vi "Main.vi"(8 "error in":errorcluster, 11 "Controller in":refnum<class "Controller.lvclass">) -> (0 "error out":errorcluster, 3 "Controller out":refnum<class "Controller.lvclass">)   [LabVIEW 2024, in "Controller.lvclass"]
doc: "The <b>Queued Message Handler</b> of the Worker that owns this VI."
uses:
  Controller.lvclass
  Controller.lvclass/Controller.ctl
  Initialization Data.ctl
  Response Cases.ctl
  <vilib>/addons/_Workers/Library/Case Label.ctl
  <vilib>/addons/_Workers/Library/Workers.lvlib
  rqp_Receive CPU Precent.ctl
  CPU Percent/CPU Percent.lvclass
  Place Temperature/Place Temperature.lvclass
  Place Temperature/rqp_Set Place.ctl
  rqp_Receive Temperature.ctl
  Report/Report.lvclass
  Report/rqp_Receive Log Interval.ctl
  rwr_Get Actual Data Reply.ctl
  C:/Program Files (x86)/National Instruments/LabVIEW 2024/vi.lib/addons/_Workers/Library/Classes/Worker/Worker.lvclass
  BEEP/BEEP.lvclass
panel:
  in  "Log Interval [ms]":i32=2000
  in  "bShowCSV":bool
  in  "Places":string(combo)="Baden, CH"
  out "Temperature":dbl(graph)
  out "Percentage":dbl(graph)
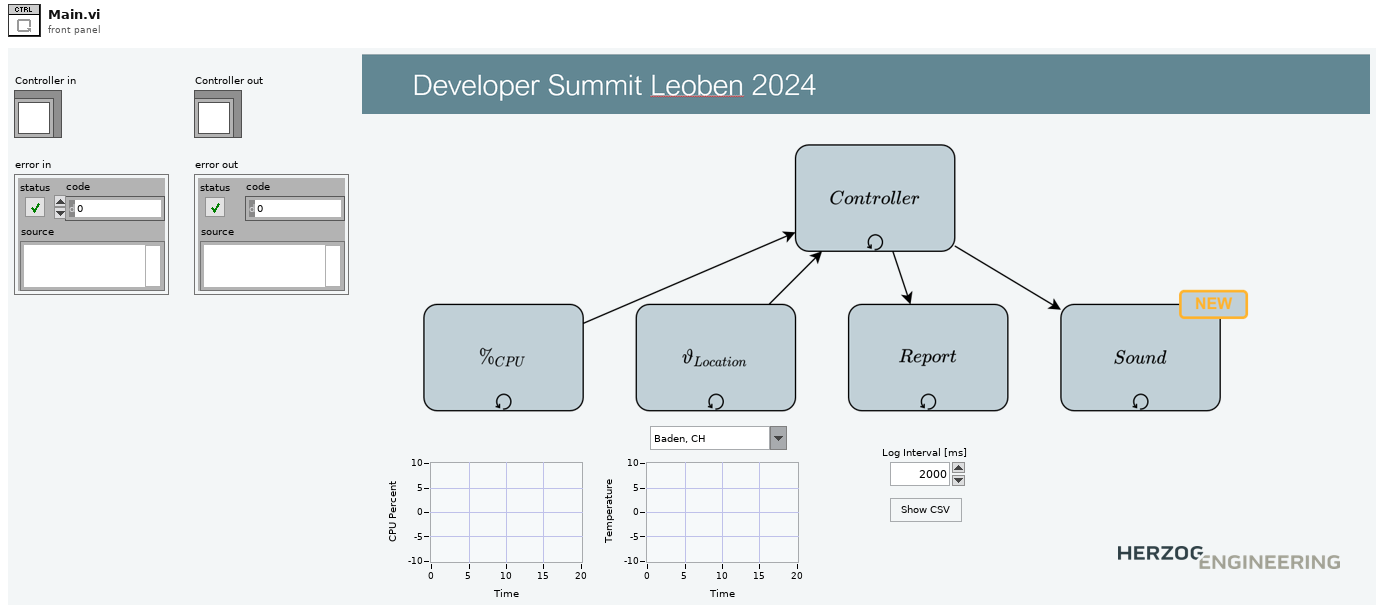
[diagram p1: front panel]
types:
  T1 = typedef "Controller.lvclass/Initialization Data.ctl" = cluster{"Response Cases":T2, "Show Frontpanel":bool}
  T2 = typedef "Controller.lvclass/Response Cases.ctl" = cluster{"Placeholder - Can be deleted":string, "Receive CPU Precent":T3}
  T3 = typedef "Workers.lvlib/Case Label.ctl" = string
  T4 = typedef "Controller.lvclass/rqp_Receive CPU Precent.ctl" = cluster{"CPU Precent":dbl}
  T5 = typedef "Controller.lvclass/rqp_Receive Temperature.ctl" = cluster{"Temperature":dbl}
  T6 = typedef "Controller.lvclass/rwr_Get Actual Data Reply.ctl" = cluster{"Temperature [°C]":dbl, "CPU [%]":dbl, "Place":string, "Timestamp":timestamp}
  T7 = typedef "Place Temperature.lvclass/rqp_Set Place.ctl" = cluster{"Place":string}
  T8 = typedef "Report.lvclass/rqp_Receive Log Interval.ctl" = cluster{"Interval [ms]":i32}
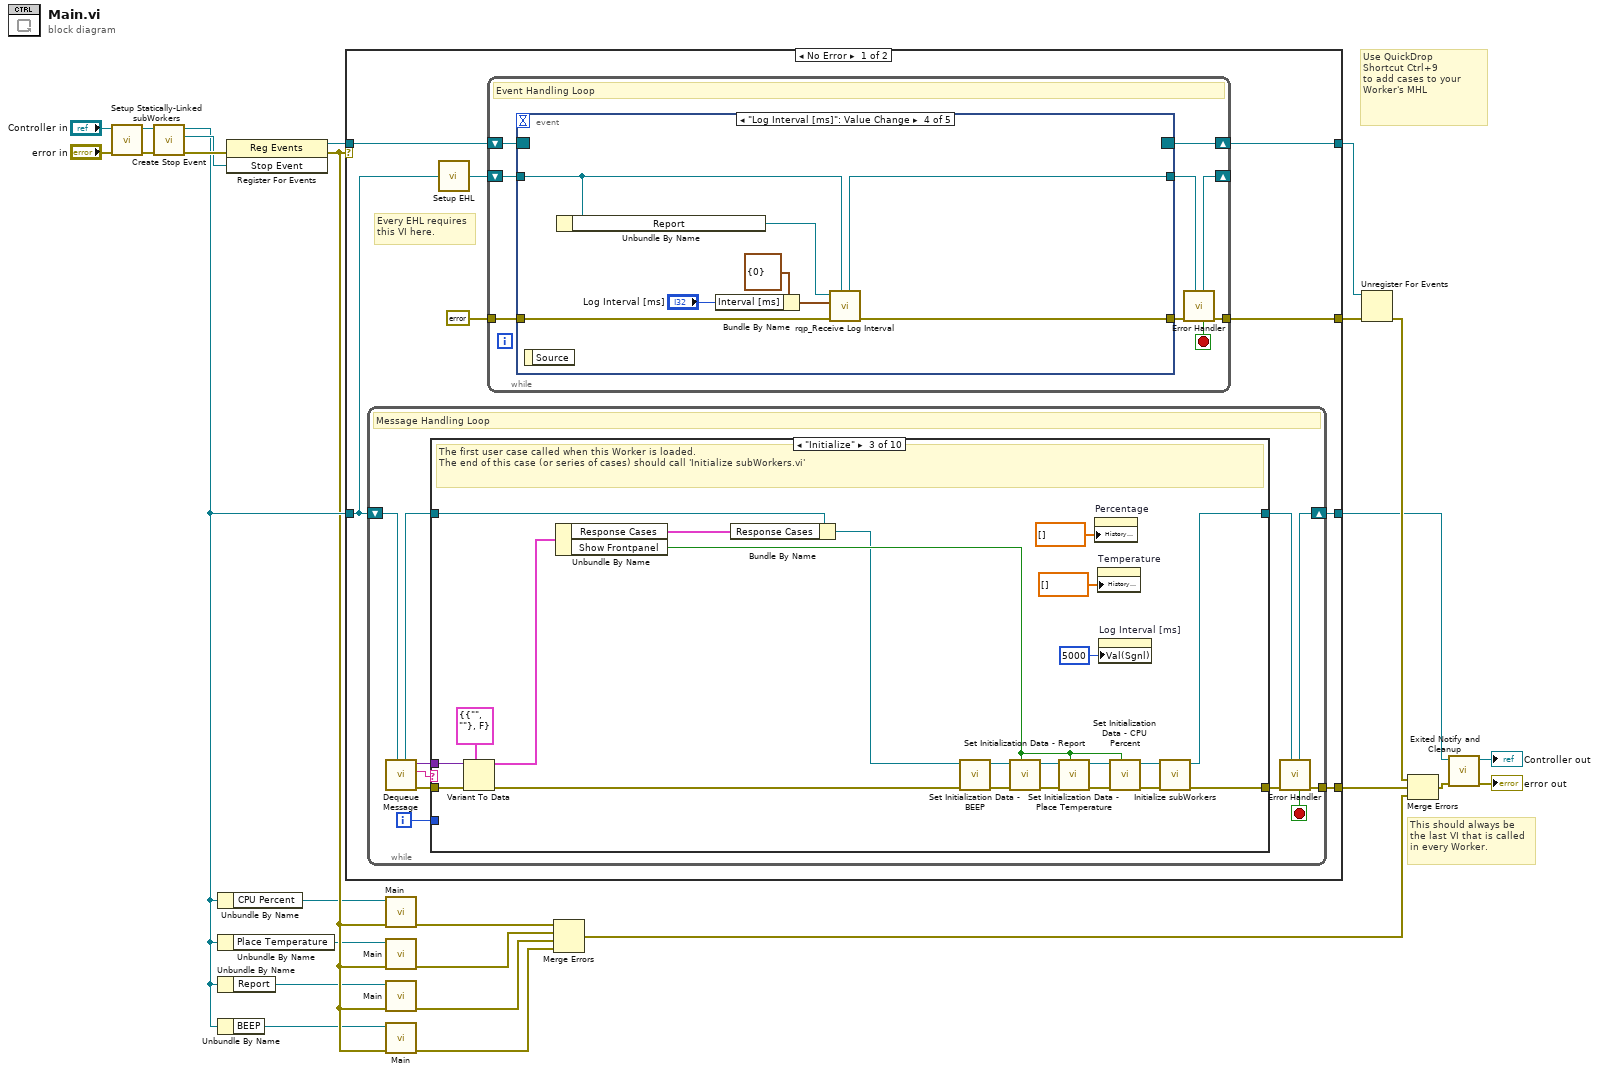
[diagram p0: block diagram]
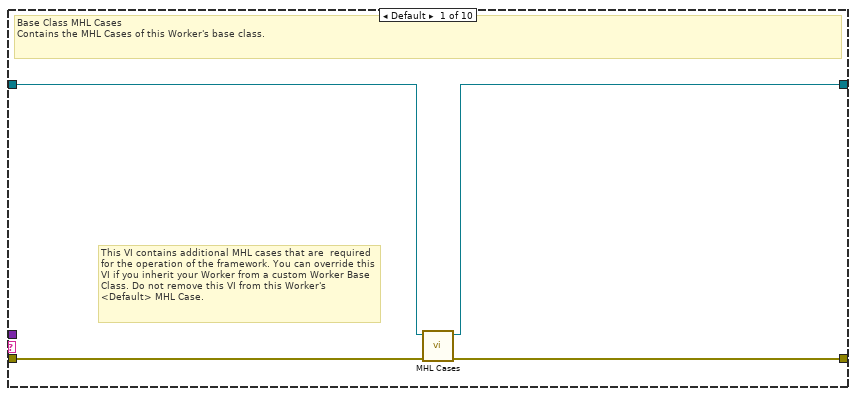
[diagram p2: hidden frame]
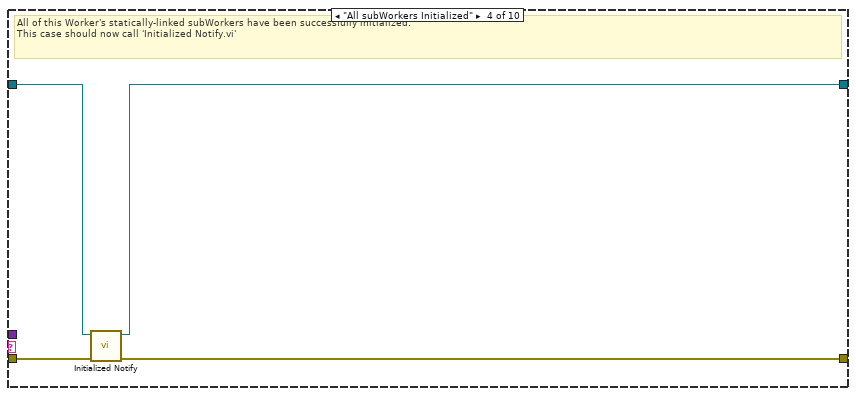
[diagram p4: hidden frame]
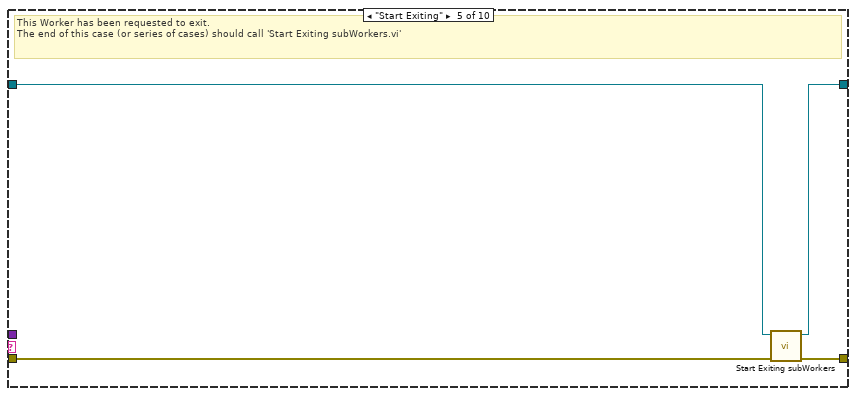
[diagram p5: hidden frame]
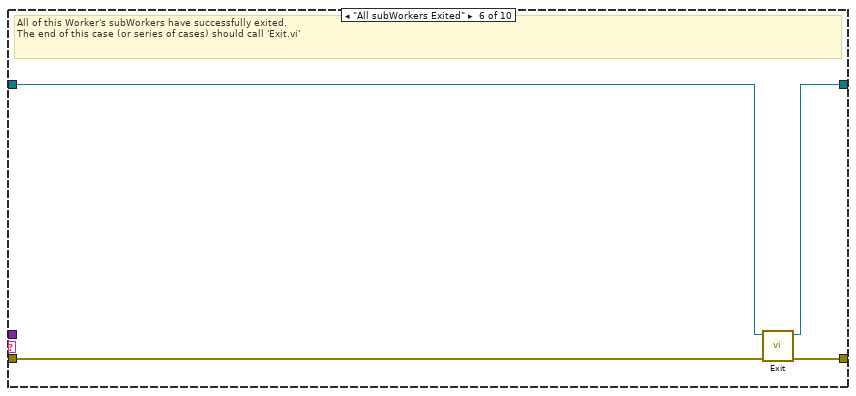
[diagram p6: hidden frame]
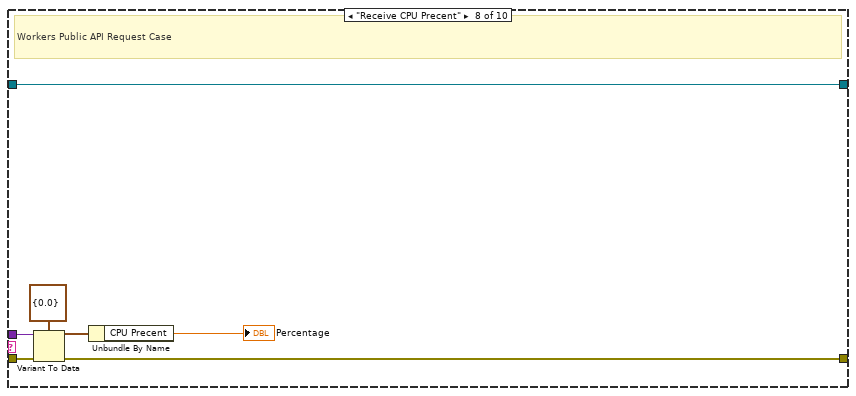
[diagram p8: hidden frame]
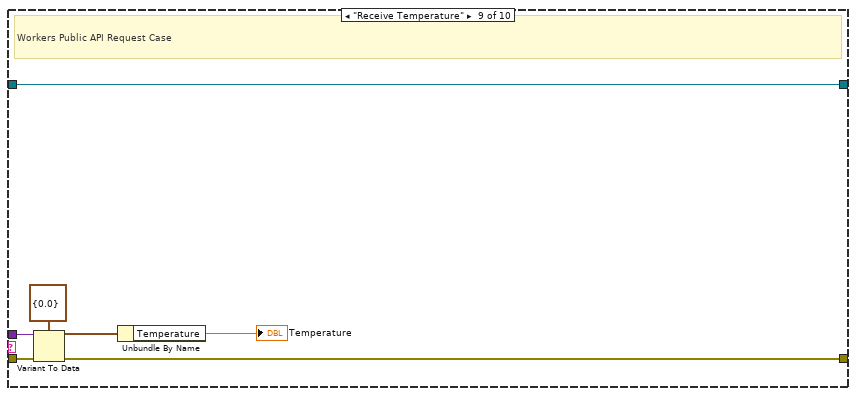
[diagram p9: hidden frame]
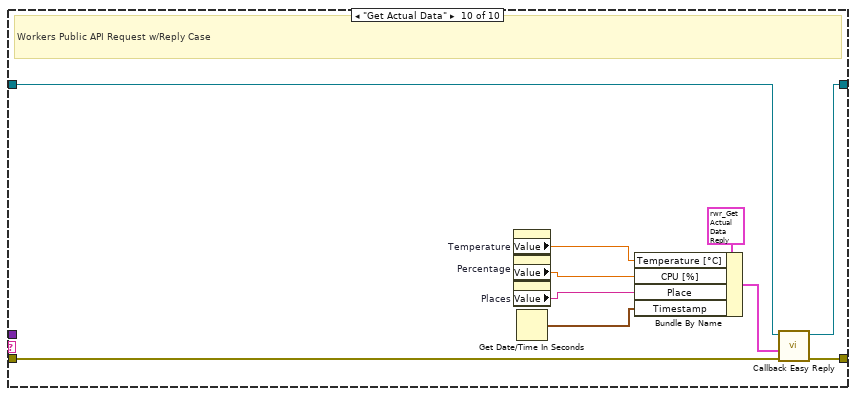
[diagram p10: hidden frame]
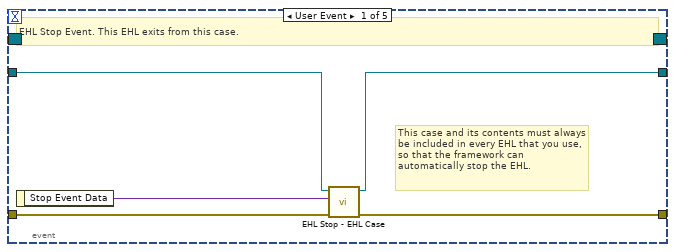
[diagram p11: hidden frame]
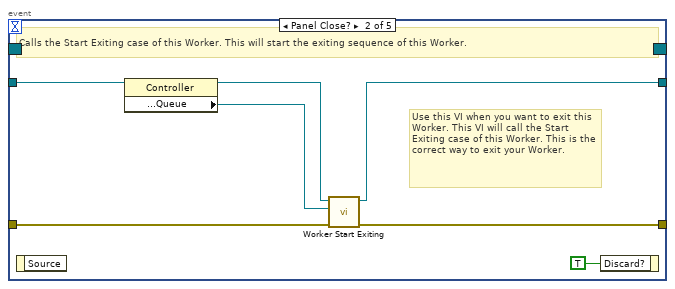
[diagram p12: hidden frame]
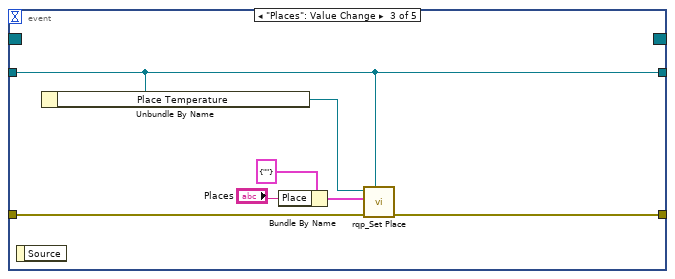
[diagram p13: hidden frame]
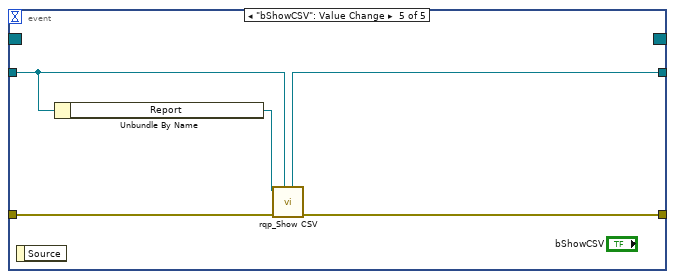
[diagram p14: hidden frame]
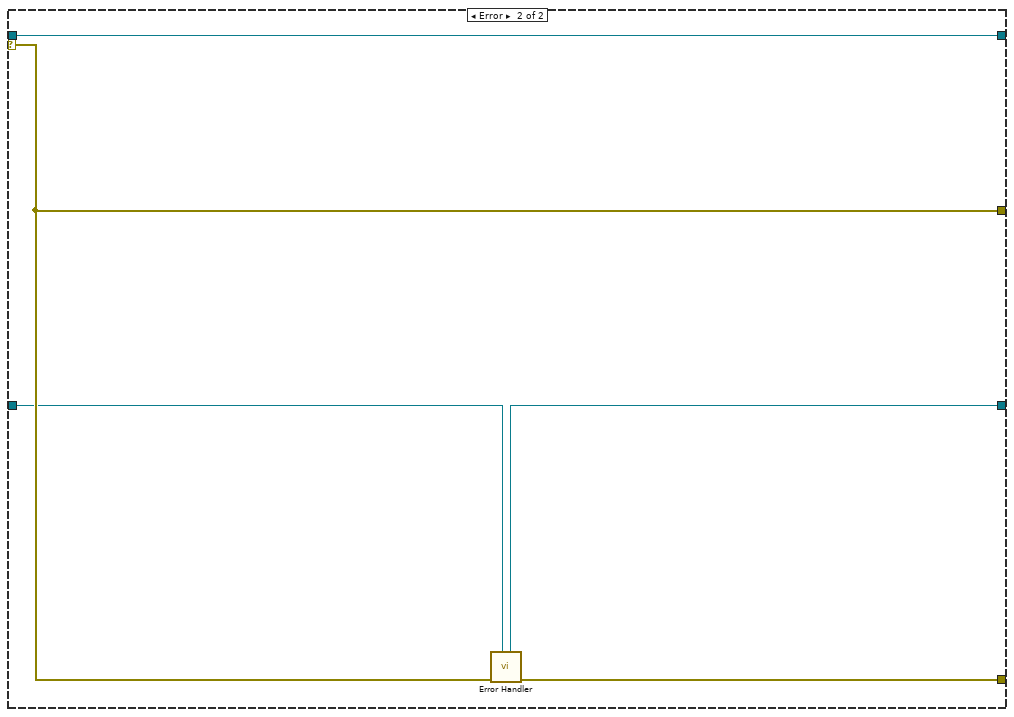
[diagram p15: hidden frame]
diagram:
  # "Use QuickDrop\nShortcut Ctrl+9\nto add cases to your\nWorker's MHL"
  # "This should always be the last VI that is called in every Worker."
  n1 = call "Setup Statically-Linked subWorkers.vi"("error in"="error in", "Controller in"="Controller in") -> ("error out"=w12:errorcluster, "Controller out"=w10:refnum<class "Controller.lvclass">)  [unwired: 8 in]
  n2 = call-dynamic "Create Stop Event.vi"("error in"=w12, "Worker"=w10) -> ("error out"=w21:errorcluster, "Stop Event"=w18:refnum<user-event>, "Worker out"=w15:refnum<class "Controller.lvclass">)  [unwired: 7 in]
  n3 = Unbundle By Name(w15) -> ("CPU Percent"=w7:refnum<class "CPU Percent.lvclass">)
  n4 = Unbundle By Name(w15) -> ("Place Temperature"=w5:refnum<class "Place Temperature.lvclass">)
  n5 = Unbundle By Name(w15) -> ("Report"=w3:refnum<class "Report.lvclass">)
  n6 = Unbundle By Name(w15) -> ("BEEP"=w1:refnum<class "BEEP.lvclass">)
  n7 = register-events(error in=w21, w18) -> (reference out=w20:refnum<event-registration>, error out=w13:errorcluster)  [unwired: 1 in]
  n8 = case shown="No Error" w13 {
    tunnel: w15 -> [w29 w154]
    tunnel: [w27 w155] -> w19
    tunnel: w20 -> [w34 w156]
    tunnel: [w31 w157] -> w25
    tunnel: [w33 w156] -> w24
    tunnel: [w28 w153] -> w22
    selector: w13 -> [_ w157]
    frame No Error {
      # "Every EHL requires\nthis VI here."
      n9 = while {
        shift-right: [w43] -> w28
        shift-left: w29 -> [w45]
        tunnel: [w44] -> w27
        i -> [w36]
        stop <- w37 stop-if-true
        # "Message Handling Loop"
        n10 = call-dynamic "Dequeue Message.vi"("Worker"=w45) -> ("error out"=w42:errorcluster, "Case out"=w38:string, "Data out"=w35:variant, "Worker out"=w40:refnum<class "Controller.lvclass">)  [unwired: 6 in, 1 out]
        n11 = case "Worker MHL Case Structure (DO NOT CHANGE LABEL NAME)" shown="\"Initialize\"" w38 {
          tunnel: w42 -> [w49 w50 w71 w75 w78 w85 w87 w93 w101 w103]
          tunnel: [w48 w50 w73 w74 w81 w84 w87 w92 w100 w111] -> w41
          tunnel: w40 -> [w47 w51 w70 w77 w79 w83 w86 w94 w95 w102]
          tunnel: [w46 w51 w72 w76 w80 w82 w86 w94 w95 w110] -> w39
          tunnel: w36 -> [_ _ _ _ _ _ _ _ _ _]
          tunnel: w35 -> [_ _ w68 _ _ _ _ w90 w98 _]
          frame Default {
            # "This VI contains additional MHL cases that are  required for the operation of the framework. You can override this VI if you inherit your Worker from a custom Worker Base Class. Do not remove this VI from this Worker's <Default> MHL Case."
            # "Base Class MHL Cases\nContains the MHL Cases of this Worker's base class."
            n12 = call-dynamic "MHL Cases.vi"("error in"=w49, "Worker in"=w47) -> ("error out"=w48:errorcluster, "Worker out"=w46:refnum<class "Controller.lvclass">)  [unwired: 8 in]
          }
          frame "------------ FRAMEWORK CASES -----------" {
            # "Start of Workers Framework Cases"
          }
          frame "Initialize" {
            # "The first user case called when this Worker is loaded.\nThe end of this case (or series of cases) should call 'Initialize subWorkers.vi'"
            n13 = Variant To Data(error in=w71, type=T1 {"Response Cases"={"Placeholder - Can be deleted"="", "Receive CPU Precent"=""}, "Show Frontpanel"=FALSE} ("Initialization Data"), Variant=w68) -> (data=w67:T1, error out=w69:errorcluster)
            n14 = Unbundle By Name(w67) -> ("Response Cases"=w66:T2, "Show Frontpanel"=w54:bool)
            n15 = Bundle By Name(cluster=w70, "Response Cases"=w66) -> (w52:refnum<class "Controller.lvclass">)
            n16 = call "Set Initialization Data - BEEP.vi"("error in"=w69, "Controller in"=w52) -> ("error out"=w56:errorcluster, "Controller out"=w55:refnum<class "Controller.lvclass">)  [unwired: 8 in]
            n17 = call "Set Initialization Data - Report.vi"("Show Frontpanel"=w54, "error in"=w56, "Controller in"=w55) -> ("error out"=w58:errorcluster, "Controller out"=w57:refnum<class "Controller.lvclass">)  [unwired: 7 in]
            n18 = call "Set Initialization Data - Place Temperature.vi"("Show Frontpanel"=w54, "error in"=w58, "Controller in"=w57) -> ("error out"=w62:errorcluster, "Controller out"=w61:refnum<class "Controller.lvclass">)  [unwired: 7 in]
            n19 = property on="Percentage" class="WFChart (strict)"("History Data"=dbl[] []) -> ()  [unwired: 2 in, 2 out]
            n20 = property on="Temperature" class="WFChart (strict)"("History Data"=dbl[] []) -> ()  [unwired: 2 in, 2 out]
            n21 = property on="Log Interval [ms]" class="DigNum (strict)"("Val(Sgnl)"=5000 ("Value (Signaling)")) -> ()  [unwired: 2 in, 2 out]
            n22 = call "Set Initialization Data - CPU Percent.vi"("Show Frontpanel"=w54, "error in"=w62, "Controller in"=w61) -> ("error out"=w64:errorcluster, "Controller out"=w63:refnum<class "Controller.lvclass">)  [unwired: 7 in]
            n23 = call-dynamic "Initialize subWorkers.vi"("error in"=w64, "Worker"=w63) -> ("error out"=w73:errorcluster, "dup Worker out"=w72:refnum<class "Controller.lvclass">)  [unwired: 8 in]
          }
          frame "All subWorkers Initialized" {
            # "All of this Worker's statically-linked subWorkers have been successfully initialized.\nThis case should now call 'Initialized Notify.vi'"
            n24 = call-dynamic "Initialized Notify.vi"("error in"=w75, "Worker"=w77) -> ("error out"=w74:errorcluster, "dup Worker out"=w76:refnum<class "Controller.lvclass">)  [unwired: 8 in]
          }
          frame "Start Exiting" {
            # "This Worker has been requested to exit. \nThe end of this case (or series of cases) should call 'Start Exiting subWorkers.vi'"
            n25 = call-dynamic "Start Exiting subWorkers.vi"("error_in"=w78, "Worker"=w79) -> ("error out"=w81:errorcluster, "dup Worker out"=w80:refnum<class "Controller.lvclass">)  [unwired: 8 in]
          }
          frame "All subWorkers Exited" {
            # "All of this Worker's subWorkers have successfully exited. \nThe end of this case (or series of cases) should call 'Exit.vi'"
            n26 = call-dynamic "Exit.vi"("error_in"=w85, "Worker"=w83) -> ("error out"=w84:errorcluster, "dup Worker out"=w82:refnum<class "Controller.lvclass">)  [unwired: 8 in]
          }
          frame "------------- PUBLIC API CASES -------------" {
            # "Start of Workers Public API Cases"
          }
          frame "Receive CPU Precent" {
            # "Workers Public API Request Case"
            n27 = Variant To Data(error in=w93, type=T4 {"CPU Precent"=0.0} ("Data"), Variant=w90) -> (data=w89:T4, error out=w92:errorcluster)
            n28 = Unbundle By Name(w89) -> ("CPU Precent"=→"Percentage":dbl)
          }
          frame "Receive Temperature" {
            # "Workers Public API Request Case"
            n29 = Variant To Data(error in=w101, type=T5 {"Temperature"=0.0} ("Data"), Variant=w98) -> (data=w97:T5, error out=w100:errorcluster)
            n30 = Unbundle By Name(w97) -> ("Temperature"=→"Temperature":dbl)
          }
          frame "Get Actual Data" {
            # "Workers Public API Request w/Reply Case"
            n31 = property on="Temperature" class="WFChart (strict)"() -> ("Value"=w107:dbl)  [unwired: 2 in, 2 out]
            n32 = property on="Percentage" class="WFChart (strict)"() -> ("Value"=w106:dbl)  [unwired: 2 in, 2 out]
            n33 = property on="Places" class="CmbBox"() -> ("Value"=w105:string)  [unwired: 2 in, 2 out]
            n34 = Get Date/Time In Seconds() -> (seconds since 1Jan1904=w104:timestamp)
            n35 = Bundle By Name(cluster=T6 {"Temperature [°C]"=0.0, "CPU [%]"=0.0, "Place"="", "Timestamp"=timestamp(0 s since 1904-01-01)} ("Reply Data"), "Temperature [°C]"=w107, "CPU [%]"=w106, "Place"=w105, "Timestamp"=w104) -> (w108:T6)
            n36 = call-dynamic "Callback Easy Reply.vi"("error in"=w103, "Data"=w108, "Worker"=w102) -> ("error out"=w111:errorcluster, "dup Worker out"=w110:refnum<class "Controller.lvclass">)  [unwired: 7 in]
          }
        }
        n37 = call-dynamic "Error Handler.vi"("Worker"=w39, "error_in"=w41) -> ("error out"=w44:errorcluster, "Stop Loop"=w37:bool, "Worker out"=w43:refnum<class "Controller.lvclass">)  [unwired: 7 in]
      }
      n38 = call-dynamic "Setup EHL.vi"("Worker"=w29) -> ("Worker out"=w30:refnum<class "Controller.lvclass">)  [unwired: 14 in]
      n39 = while "Event Handling Loop" {
        shift-right: [w120] -> w33
        shift-left: w34 -> [w119]
        tunnel: [w115] -> w31
        tunnel: errorcluster {"status"=FALSE, "code"=0, "source"=""} ("error constant") -> [w117]
        shift-right: [w113] -> _
        shift-left: w30 -> [w118]
        stop <- w112 stop-if-true
        # "Event Handling Loop"
        n40 = event shown="[3] \"Log Interval [ms]\": Value Change" {
          selector: w119 -> [_ _ _ _ _]
          dyn-events: [_ _ _ _ _] -> w120
          timeout: _ -> [_ _ _ _ _]
          tunnel: [w124 w131 w135 w146 w151] -> w116
          tunnel: w117 -> [w125 w130 w136 w147 w152]
          tunnel: w118 -> [w123 w129 w134 w144 w149]
          tunnel: [w122 w128 w134 w145 w150] -> w114
          event User Event {
            # "This case and its contents must always be included in every EHL that you use, so that the framework can automatically stop the EHL."
            # "EHL Stop Event. This EHL exits from this case."
            n41 = event-data() -> ("Stop Event Data"=w121:variant)  [unwired: 1 in]
            n42 = call-dynamic "EHL Stop - EHL Case.vi"("error in"=w125, "Stop Event Data"=w121, "Worker"=w123) -> ("error out"=w124:errorcluster, "Worker out"=w122:refnum<class "Controller.lvclass">)  [unwired: 7 in]
          }
          event Panel Close? {
            # "Use this VI when you want to exit this Worker. This VI will call the Start Exiting case of this Worker. This is the correct way to exit your Worker."
            # "Calls the Start Exiting case of this Worker. This will start the exiting sequence of this Worker."
            n43 = event-data() -> ()  [unwired: 1 in, 1 out]
            n44 = property class="Controller"(reference=w129) -> (reference out=w127:refnum<class "Controller.lvclass">, "Accessors:Read:Public API:Queue"=w126:refnum<class "Message Queue.lvclass">)  [unwired: 1 in, 1 out]
            n45 = call-dynamic "Worker Start Exiting.vi"("error_in"=w130, "Message Queue"=w126, "Worker"=w127) -> ("error out"=w131:errorcluster, "dup Worker out"=w128:refnum<class "Controller.lvclass">)  [unwired: 7 in]
            n46 = event-data ("Event Filter Node")("Discard?"=TRUE) -> ()  [unwired: 1 in, 1 out]
          }
          event "Places": Value Change {
            n47 = event-data() -> ()  [unwired: 1 in, 1 out]
            n48 = Unbundle By Name(w134) -> ("Place Temperature"=w133:refnum<class "Place Temperature.lvclass">)
            n49 = Bundle By Name(cluster=T7 {"Place"=""} ("Data in"), "Place"="Places") -> (w138:T7)
            n50 = call "rqp_Set Place.vi"("Caller in"=w134, "error in"=w136, "Data in"=w138, "Place Temperature in"=w133) -> ("error out"=w135:errorcluster)  [unwired: 5 in, 2 out]
          }
          event "Log Interval [ms]": Value Change {
            n51 = event-data() -> ()  [unwired: 1 in, 1 out]
            n52 = Unbundle By Name(w144) -> ("Report"=w143:refnum<class "Report.lvclass">)
            n53 = Bundle By Name(cluster=T8 {"Interval [ms]"=0} ("Data in"), "Interval [ms]"="Log Interval [ms]") -> (w142:T8)
            n54 = call "rqp_Receive Log Interval.vi"("Caller in"=w144, "error in"=w147, "Data in"=w142, "Report in"=w143) -> ("error out"=w146:errorcluster, "dup Caller out"=w145:refnum<class "Controller.lvclass">)  [unwired: 5 in, 1 out]
          }
          event "bShowCSV": Value Change {
            n55 = event-data() -> ()  [unwired: 1 in, 1 out]
            n56 = Unbundle By Name(w149) -> ("Report"=w148:refnum<class "Report.lvclass">)
            n57 = call "rqp_Show CSV.vi"("Caller in"=w149, "error in"=w152, "Report in"=w148) -> ("error out"=w151:errorcluster, "dup Caller out"=w150:refnum<class "Controller.lvclass">)  [unwired: 6 in, 1 out]
          }
        }
        n58 = call-dynamic "Error Handler.vi"("Worker"=w114, "error_in"=w116) -> ("error out"=w115:errorcluster, "Stop Loop"=w112:bool, "Worker out"=w113:refnum<class "Controller.lvclass">)  [unwired: 7 in]
      }
    }
    frame Error {
      n59 = call-dynamic "Error Handler.vi"("Worker"=w154, "error_in"=w157) -> ("error out"=w155:errorcluster, "Worker out"=w153:refnum<class "Controller.lvclass">)  [unwired: 7 in, 1 out]
    }
  }
  n60 = call-dynamic "Main.vi"("error in"=w13, "CPU Percent in"=w7) -> ("error out"=w9:errorcluster)  [unwired: 8 in, 1 out]
  n61 = call-dynamic "Main.vi"("error in"=w13, "CPU Percent in"=w5) -> ("error out"=w6:errorcluster)  [unwired: 8 in, 1 out]
  n62 = call-dynamic "Main.vi"("error in"=w13, "Report in"=w3) -> ("error out"=w4:errorcluster)  [unwired: 8 in, 1 out]
  n63 = call-dynamic "Main.vi"("error in"=w13, "BEEP in"=w1) -> ("error out"=w2:errorcluster)  [unwired: 8 in, 1 out]
  n64 = Merge Errors(w9, w6, w4, w2) -> (w8:errorcluster)
  n65 = Unregister For Events(event registration refnum=w24, error in=w25) -> (error out=w26:errorcluster)
  n66 = Merge Errors(w26, w19, w8) -> (w23:errorcluster)
  n67 = call-dynamic "Exited Notify and Cleanup.vi"("error_in"=w23, "Worker"=w22) -> ("error out"=→"error out":errorcluster, "dup Worker out"=→"Controller out":refnum<class "Controller.lvclass">)  [unwired: 8 in]
